vi "remove channel from active array_wwarning.vi"(1 "line to remove":u32, 2 "line array in":u32[](array[numeric])) -> (0 "line array out":u32[](array[numeric]))   [LabVIEW 2013]
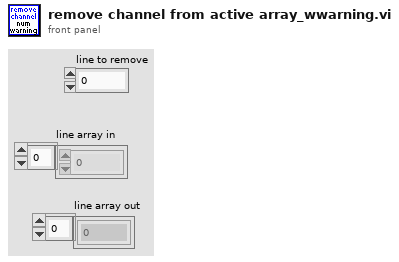
[diagram p1: front panel]
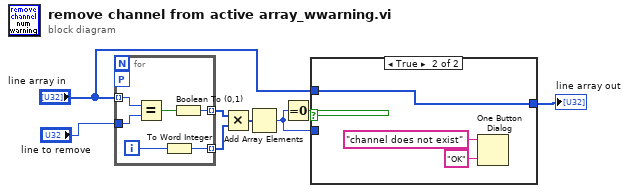
[diagram p0: block diagram]
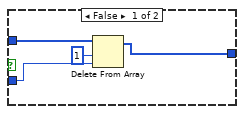
[diagram p2: hidden frame]
diagram:
  n1 = for {
    workers-P: _ -> [_]
    tunnel: "line array in" -> [w13] mode=indexing
    tunnel: "line to remove" -> [w14]
    tunnel: [w9] -> w3 mode=indexing
    tunnel: [w10] -> w4 mode=indexing
    i -> [w12]
    n2 = Equal?(x=w13, y=w14) -> (x = y?=w11:bool)
    n3 = To Word Integer(number=w12) -> (16bit integer=w9:i16)
    n4 = Boolean To (0,1)(Boolean=w11) -> (0, 1=w10:i16)
  }
  n5 = Multiply(x=w4, y=w3) -> (x*y=w2:i16[])
  n6 = Add Array Elements(numeric array=w2) -> (sum=w1:i16)
  n7 = Equal To 0?(x=w1) -> (x = 0?=w8:bool)
  n8 = case shown="True" w8 {
    tunnel: "line array in" -> [w18 w21]
    tunnel: [w15 w21] -> w5
    tunnel: w1 -> [w17 _]
    frame False {
      n9 = Delete From Array(array=w18, length=1, index=w17) -> (array with subset deleted=w15:u32[])  [unwired: 1 out]
    }
    frame True {
      n10 = One Button Dialog(message="channel does not exist", button name ("OK")="OK") -> ()  [unwired: 1 out]
    }
  }
  "line array out" <- w5
